vi "Dashboard Main.vi"() -> ()   [LabVIEW 2016]
uses:
  <vilib>/Utility/miscctls.llb/LVRowAndColumnTypeDef.ctl
  <vilib>/event_ctls.llb/eventvkey.ctl
  <vilib>/Rock Robotics/Network Tables/NT Read Numeric Array.vi
  <vilib>/Rock Robotics/WPI/Dashboard/WPI_DashboardLogging Global.vi
panel:
  in  "Camera Settings Right":T1={"Frame Rate"=30, "Compression"=30, "Size"=1, "DB Camera Config"=FALSE} {"Frame Rate" scale=1.0..30.0; "Compression" scale=100.0..-1.0; "Size" items=["640x480", "320x240", "160x120"]}
  in  "Camera Name Right":string(combo)="No Camera Selection"
  out "Camera Info":cluster{"Mbps LED":bool, "Mbps":dbl, "fps":dbl} {"fps" format="%#.1g"; "Mbps" format="%#.1g"}
  in  "Camera Settings":T1={"Frame Rate"=30, "Compression"=30, "Size"=1, "DB Camera Config"=FALSE} {"Frame Rate" scale=1.0..30.0; "Compression" scale=100.0..-1.0; "Size" items=["640x480", "320x240", "160x120"]}
  in  "TCP":refnum<k5>
  in  "Rec Mode":enum32{"Stop", "Record", "Playback"}(radio)
  out "Robot IP":string
  out "Image Message":string="Timeout in Camera Communications"
  in  "Dashboard Tab":T2(tab)
  in  "Select Auto":string(combo)="Select Autonomous ..."
  out "NT Connection":bool
  out "MotorChart R":cluster{"Numeric":dbl, "Numeric":dbl}(graph)
  out "MotorChart L":cluster{"Numeric":dbl, "Numeric":dbl}(graph)
  out "MotorSliders R":cluster{"MotorSlide1":dbl, "MotorSlide2":dbl} {"MotorSlide2" scale=-1.0..1.0 scale format="%#_2e"; "MotorSlide1" scale=-1.0..1.0 scale format="%#_2e"}
  out "MotorSliders L":cluster{"MotorSlide1":dbl, "MotorSlide2":dbl} {"MotorSlide2" scale=-1.0..1.0 scale format="%#_2e"; "MotorSlide1" scale=-1.0..1.0 scale format="%#_2e"}
  out "Gyro":dbl(knob) scale=0.0..360.0
  out "JS1 Z":dbl(slide) scale=-1.0..1.0 scale format="%#_2e"
  out "JS1 Graph":cluster{"X":dbl, "Y":dbl}[](graph)
  out "JS1 Buttons":T3
  out "JS2 Z":dbl(slide) scale=-1.0..1.0 scale format="%#_2e"
  out "JS2 Graph":cluster{"X":dbl, "Y":dbl}[](graph)
  out "JS2 Buttons":T3
  out "Mode":T4(ring)=enum."Auto Disabled"
  out "Camera Image Right":T5(plugin-control)
  in  "DB/String 9":string
  in  "DB/String 8":string
  in  "DB/String 7":string
  in  "DB/String 6":string
  in  "DB/String 5":string
  in  "DB/String 4":string
  in  "DB/String 3":string
  in  "DB/String 2":string
  in  "DB/String 1":string
  in  "DB/String 0":string
  in  "DB/Slider 0":dbl(slide) scale=0.0..5.0
  in  "DB/Slider 1":dbl(slide) scale=0.0..5.0
  in  "DB/Slider 2":dbl(slide) scale=0.0..5.0
  in  "DB/Slider 3":dbl(slide) scale=0.0..5.0
  out "DB/LED 3":bool
  out "DB/LED 2":bool
  out "DB/LED 1":bool
  out "DB/LED 0":bool
  in  "DB/Button 3":bool
  in  "DB/Button 2":bool
  in  "DB/Button 1":bool
  in  "DB/Button 0":bool caption="New Name"
  in  "JoystickModes":u16(ring)=3 items=["Arcade Joystick", "Tank", "Xbox top", "Xbox Right"]
  in  "Test Slider":dbl(slide) scale=0.0..100.0 scale format="%#_3g"
  in  "On/Off":bool caption="Solenoid"
  in  "Test Name":u16(ring) items=["Select the test to run..."]
  in  "Test Tree":string(tree)
  in  "Motor":cluster{"Value":dbl, "Enable":bool} {"Value" scale=-1.0..1.0 scale format="%#_3g"}
  out "Progress":T6 {"Test Progress" scale=0.0..100.0}
  in  "Rev/Fwd":cluster{"Forward":bool, "Reverse":bool}
  in  "Test Ring":u16(ring) items=["Monochrome", "Color"]
  out "Cmd Status":string
  in  "Execute Command":bool
  in  "Command Params":string[][](table)
  in  "Command Selection":i32(listbox)
  in  "CheckList":i32(listbox)
  out "Tree":string(tree)
  out "Camera Image":T5(plugin-control)
  out "Background":bool
  in  "Camera Name":string(combo)="No Camera Selection"
  # "HW"
  # "HW"
  # "Joysticks"
  # "Drive Motors"
  # "Front"
  # "Right"
  # "Left"
  # "Back"
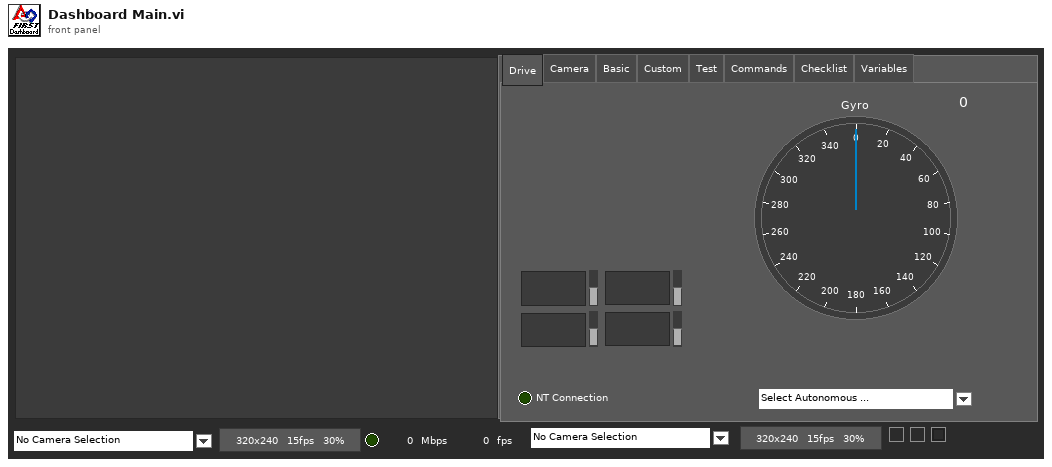
[diagram p1: front panel]
types:
  T1 = cluster{"Frame Rate":i32, "Compression":i32, "Size":u16, "DB Camera Config":bool}
  T2 = enum32{"Drive", "Camera", "Basic", "Custom", "Test", "Commands", "Checklist", "Variables"}
  T3 = cluster{bool, bool, bool, bool, bool, bool, bool, bool, bool, bool, bool, bool}
  T4 = enum8{"Tele-Op Disabled", "Tele-Op Enabled", "Auto Disabled", "Auto Enabled", "Test Disabled", "Test Enabled", "Disconnected", "No Code", "E-Stop"}
  T5 = typedef "IMAQ Image.ctl" = refnum<image>
  T6 = cluster{"Test Progress":u8, "Test Progress Text":string}
  T7 = typedef "Image Type" = u32
  T8 = cluster{"IDs":cluster{"RPC field ID":u16, "Unique ID":u16}, "String":string}
  T9 = enum32{"Drive", "Basic", "Custom", "Test", "Checklist", "Variables"}
  T10 = cluster{"Error Strings":string, "Disable Counts":cluster{u16, u16}, "Rail Faults":cluster{u16, u16, u16}, "Robot IP":string, "DB Mode":u8, "Event Info":cluster{"Name":string, "Type":u8, "Number":u16, "Replay":u8}}
  T11 = cluster{"Storage":cluster{"Disk Free":u64, "RAM Block":u32, "RAM free":u32}, "CPU Utilization":cluster{"CPU % ISR":sgl, "CPU % Time Crit":sgl, "CPU % Timed Str":sgl, "CPU % High":sgl, "CPU % Above":sgl, "CPU % Normal":sgl, "CPU % Low":sgl}, "CAN":cluster{"% Bus Utilization":sgl, "Bus Off Cnt":u32, "TX_FIFO Full Cnt":u32, "Receive Error Cnt":u8, "Transmit Error Cnt":u8}, "HID":cluster{"HID Outputs":u32, "Rumble Low":u16, "Rumble High":u16}[]}
  T12 = cluster{"Status bits":cluster{"Test Mode":bool, "Autonomous":bool, "Enabled":bool, "Code Start":bool, "Brownout":bool, "Reserved 2":bool, "Reserved 3":bool, "E-Stop":bool}, "Code Trace":cluster{"Disabled":bool, "TeleOp":bool, "Auto":bool, "Test":bool}, "Controller Type":enum16{"unknown", "cRIO", "roboRio"}, "Code?":enum16{"unknown", "noCode", "code"}, "Battery V":dbl}
  T13 = cluster{"Control Bits":cluster{"TestMode":bool, "Autonomous":bool, "Enabled":bool, "FMS Present":bool, bool, bool, bool, "E-Stop":bool}, "Team Station ":u8, "Countdown":sgl, "Joystick Values":cluster{"Axes":dbl[], "Buttons":bool[], "POVs":i16[]}[]}
  T14 = cluster{"Axes":dbl[], "Buttons":bool[], "POVs":i16[]}[]
  T15 = cluster{"Axes":dbl[], "Buttons":bool[], "POVs":i16[]}
  T16 = cluster{"Buttons[0]":bool, "Buttons[1]":bool, "Buttons[2]":bool, "Buttons[3]":bool, "Buttons[4]":bool, "Buttons[5]":bool, "Buttons[6]":bool, "Buttons[7]":bool, "Buttons[8]":bool, "Buttons[9]":bool, "Buttons[10]":bool, "Buttons[11]":bool}
  T17 = cluster{"Camera Image":refnum<vi>, "Dashboard Tab":refnum<vi>, "Background":refnum<vi>, "Rec Mode":refnum<vi>, "Test Slider":refnum<vi>, "On/Off ":refnum<vi>, "Test Ring":refnum<vi>, "Rev/Fwd":refnum<vi>, "Test Name":refnum<vi>, "Motor":refnum<vi>, "Progress":refnum<vi>, "CheckList":refnum<vi>, "Tree":refnum<vi>, "Test Tree":refnum<vi>, "Command Params":refnum<vi>, "Command Selection":refnum<vi>, "Execute Command":refnum<vi>, "Cmd Status":refnum<vi>, "Camera Settings":refnum<vi>, "Camera Name":refnum<vi>, "Camera Info":refnum<vi>, "Camera Settings Right":refnum<vi>, "Camera Name Right":refnum<vi>, "Camera Image Right":refnum<vi>}
  T18 = cluster{"Operation":enum16{"Update", "Clear"}, "Color Box":u32}[]
  T19 = typedef "eventvkey.ctl" = enum16{"ASCII", "Enter", "Return", "Shift", "Ctrl", "Alt", "Cmd", "Opt", "Caps", "NumLock", "Clear", "Break", "Up", "Down", "Left", "Right", "Insert", "Delete", "Home", "End", "PageUp", "PageDown", "Escape", "Help", "Pause", "ScrollLock", "F1", "F2", "F3", "F4", "F5", "F6", "F7", "F8", "F9", "F10", "F11", "F12", "F13", "F14", "F15", "F16", "F17", "F18", "F19", "F20", "F21", "F22", "F23", "F24", "Play", "VolumeUp", "VolumeDown", "Mute", "Two Byte Char"}
  T20 = cluster{"Image Size":bool, "Image Type":bool, "Pixel Value":bool, "ROI Information":bool, "Zoom Factor":bool}
  T21 = cluster{"Operation":enum16{"Update", "Clear"}, "Color Box":u32}
  T22 = typedef "LVRowAndColumnTypeDef.ctl" = cluster{"Row":i32, "Column":i32}
  T23 = cluster{"Shift":bool, "Ctrl":bool, "Alt":bool, "Cmd":bool, "Opt":bool}
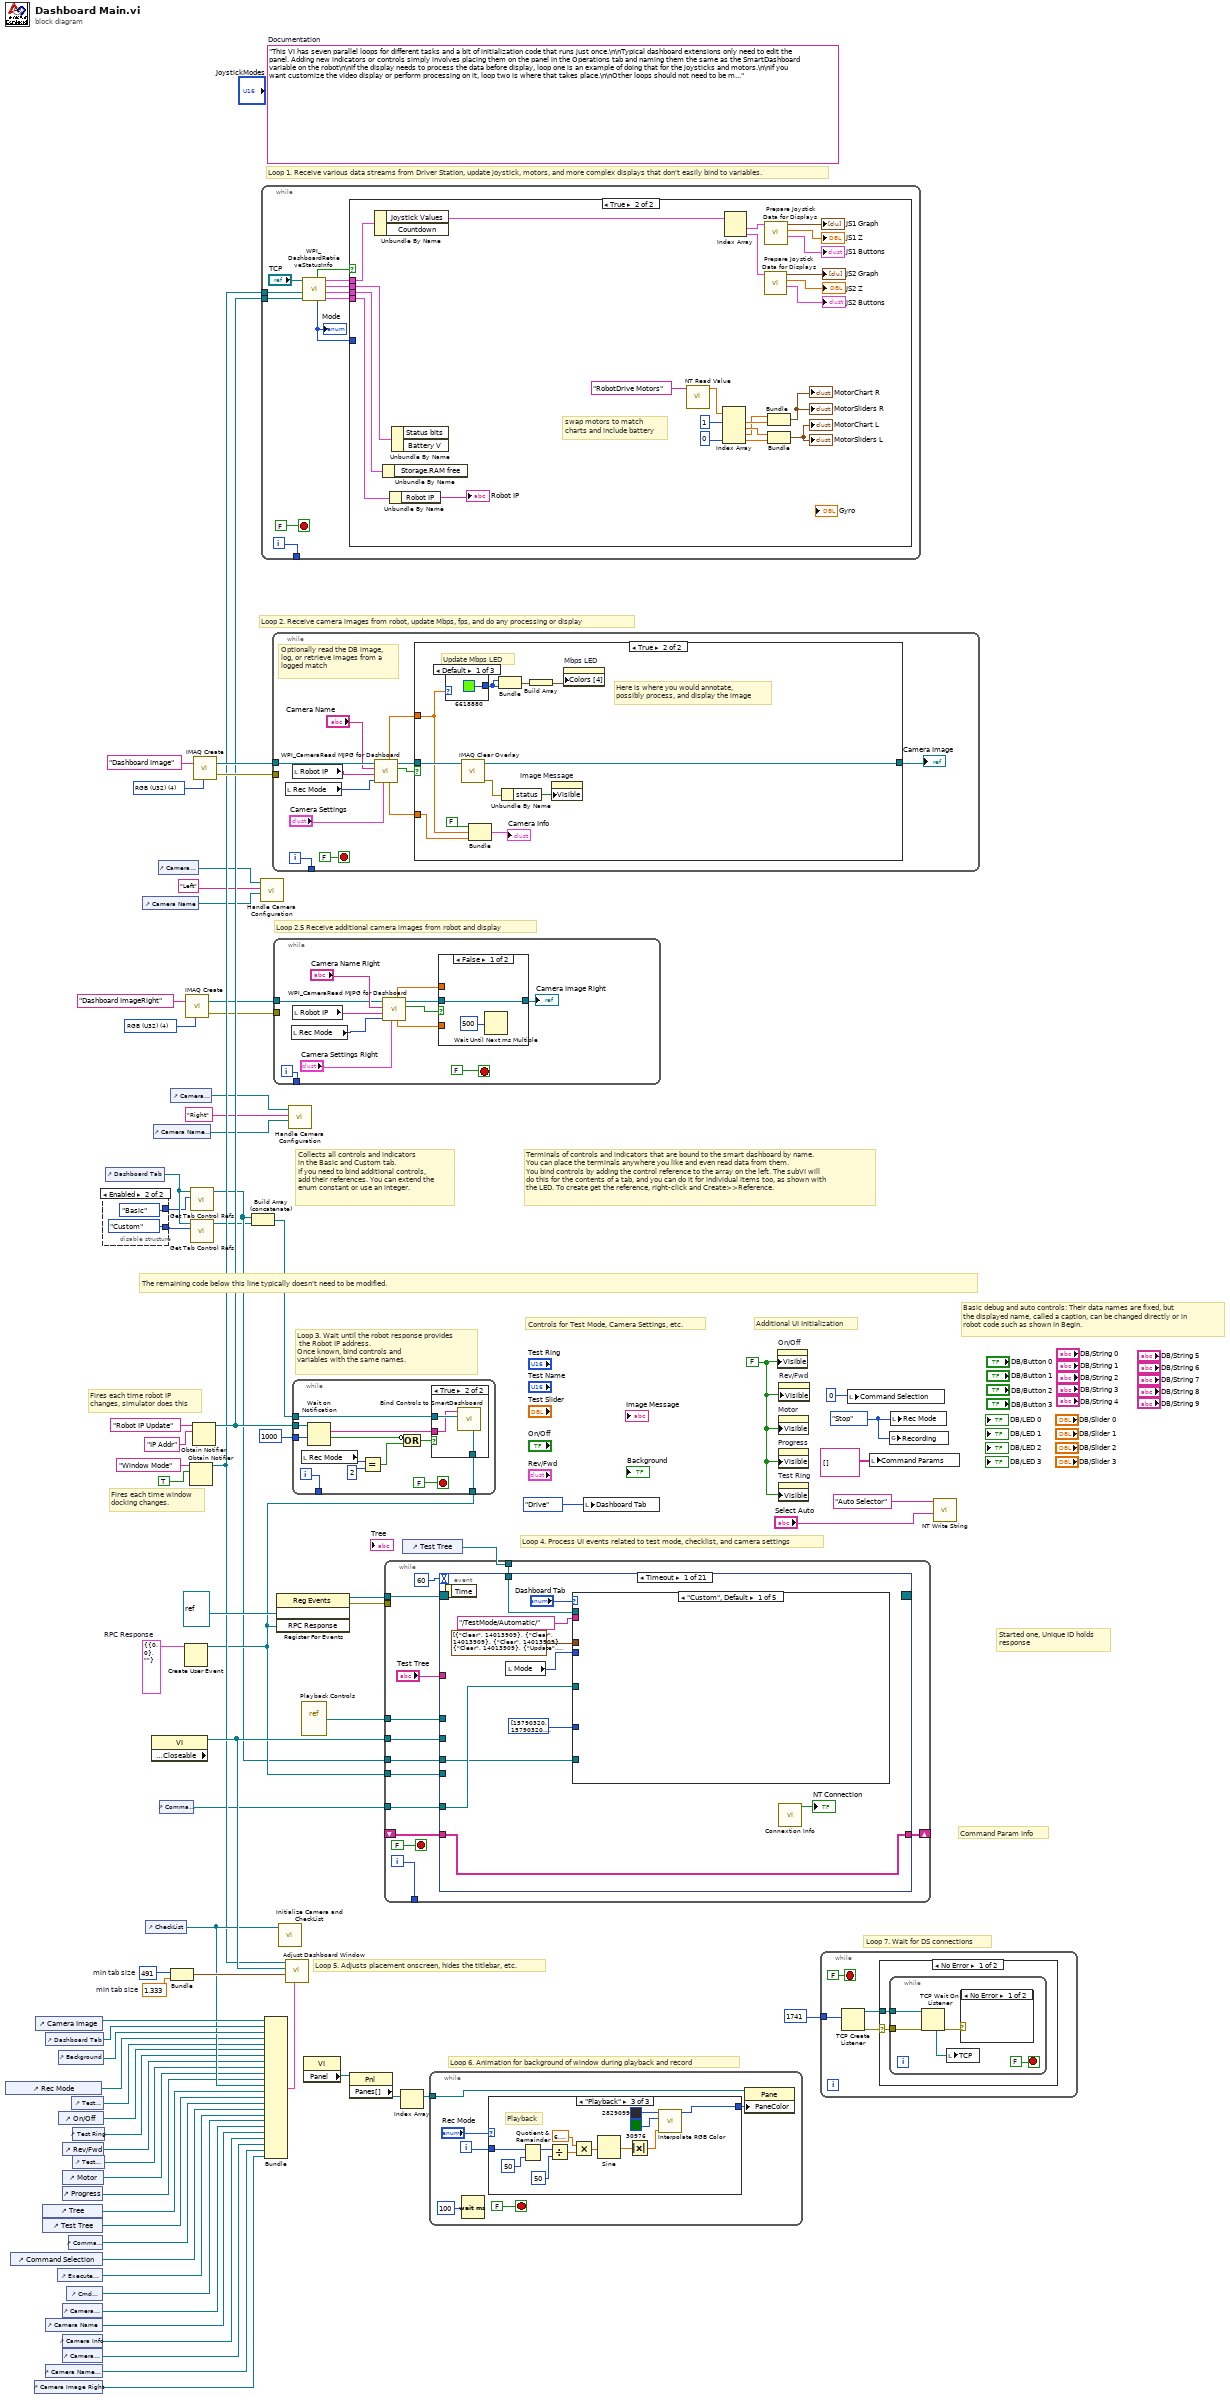
[diagram p0: block diagram]
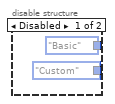
[diagram p2: hidden frame]
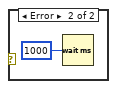
[diagram p4: hidden frame]
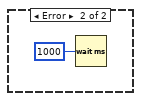
[diagram p5: hidden frame]
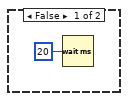
[diagram p6: hidden frame]
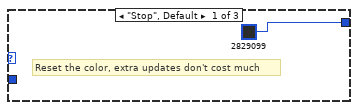
[diagram p7: hidden frame]
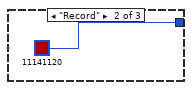
[diagram p8: hidden frame]
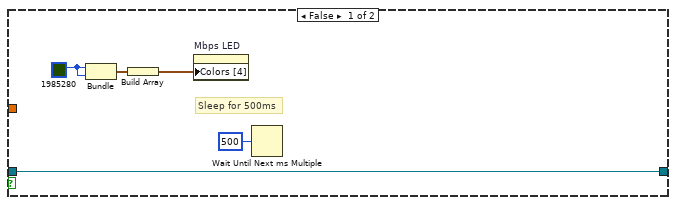
[diagram p10: hidden frame]
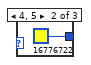
[diagram p11: hidden frame]
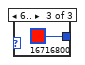
[diagram p12: hidden frame]
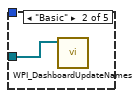
[diagram p13: hidden frame]
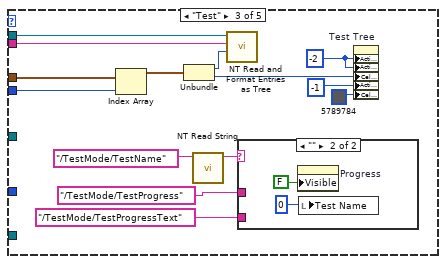
[diagram p14: hidden frame]
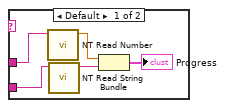
[diagram p15: hidden frame]
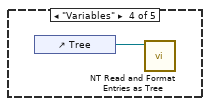
[diagram p16: hidden frame]
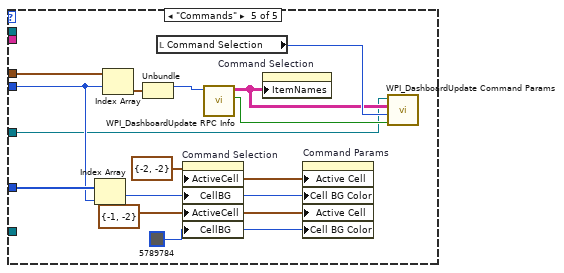
[diagram p17: hidden frame]
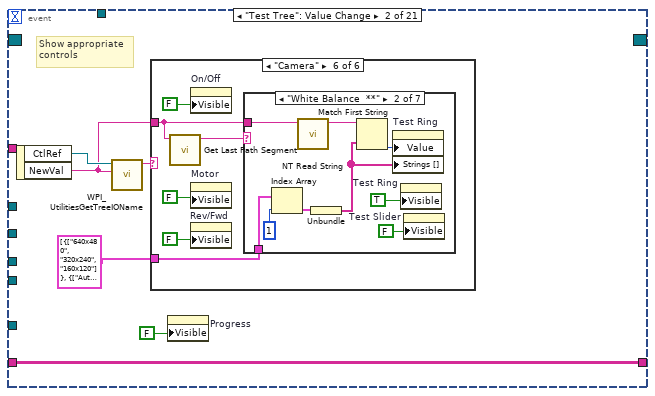
[diagram p18: hidden frame]
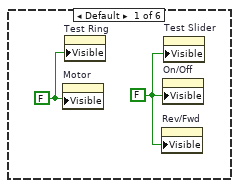
[diagram p19: hidden frame]
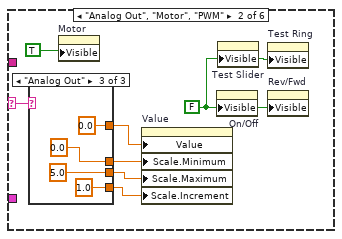
[diagram p20: hidden frame]
diagram:
  w12 = T7 4 items=["Grayscale (U8)", "Grayscale (I16)", "Grayscale (SGL)", "Complex (CSG)", "RGB (U32)", "HSL (U32)", "RGB (U64)"] ("Image Type")
  w27 = T8 {"IDs"={"RPC field ID"=0, "Unique ID"=0}, "String"=""}  # RPC Response
  w52 = 491  # min tab size
  w51 = 1.333  # min tab size
  w58 = enum32{"Stop", "Record", "Playback"}."Stop" ("Rec Mode")
  w34 = FALSE ("Visible")
  (unwired) "This VI has seven parallel loops for different tasks and a bit of initialization code that runs just once.\n\nTypical dashboard extensions only need to edit the panel. Adding new indicators or controls simply involves placing them on the panel in the Operations tab and naming them the same as the SmartDashboard variable on the robot\n\nIf the display needs to process the data before display, loop one is an example of doing that for the joysticks and motors.\n\nIf you want customize the video display or perform processing on it, loop two is where that takes place.\n\nOther loops should not need to be modified. They are pretty standard, and document the task they perform."  # Documentation
  w75 = T7 4 items=["Grayscale (U8)", "Grayscale (I16)", "Grayscale (SGL)", "Complex (CSG)", "RGB (U32)", "HSL (U32)", "RGB (U64)"] ("Image Type")
  # "Loop 2.5 Receive additional camera images from robot and display"
  # "Command Param Info"
  # "Started one, Unique ID holds\nresponse"
  # "Loop 7. Wait for DS connections"
  # "Basic debug and auto controls: Their data names are fixed, but\nthe displayed name, called a caption, can be changed directly or in\nrobot code such as shown in Begin."
  # "Controls for Test Mode, Camera Settings, etc."
  # "Additional UI Initialization"
  # "Loop 6. Animation for background of window during playback and record"
  # "Fires each time robot IP\nchanges, simulator does this"
  # "Fires each time window\ndocking changes."
  # "Collects all controls and indicators\nin the Basic and Custom tab.\nIf you need to bind additional controls,\nadd their references. You can extend the\nenum constant or use an integer."
  # "The remaining code below this line typically doesn't need to be modified."
  # "Loop 4. Process UI events related to test mode, checklist, and camera settings"
  # "Terminals of controls and indicators that are bound to the smart dashboard by name.\nYou can place the terminals anywhere you like and even read data from them.\nYou bind controls by adding the control reference to the array on the left. The subVI will\ndo this for the contents of a tab, and you can do it for individual items too, as shown with\nthe LED. To create get the reference, right-click and Create>>Reference."
  # "Loop 3. Wait until the robot response provides\n the Robot IP address.\nOnce known, bind controls and\nvariables with the same names."
  # "Loop 5. Adjusts placement onscreen, hides the titlebar, etc."
  # "Loop 1. Receive various data streams from Driver Station, update joystick, motors, and more complex displays that don't easily bind to variables."
  # "Loop 2. Receive camera images from robot, update Mbps, fps, and do any processing or display"
  n1 = control-ref of="Rec Mode"() -> (w40:refnum<vi>)
  n2 = control-ref of="Command Selection"() -> (w26:refnum<vi>)
  n3 = control-ref of="Camera Image Right"() -> (w3:refnum<vi>)
  n4 = control-ref of="Camera Image"() -> (w54:refnum<vi>)
  n5 = control-ref of="Tree"() -> (w44:refnum<vi>)
  n6 = control-ref of="Test Tree"() -> (w43:refnum<vi>)
  n7 = control-ref of="Dashboard Tab"() -> (w53:refnum<vi>)
  n8 = control-ref of="Camera Name"() -> (w17:refnum<vi>)
  n9 = control-ref of="Camera Name Right"() -> (w4:refnum<vi>)
  n10 = control-ref of="Execute Command"() -> (w28:refnum<vi>)
  n11 = control-ref of="Background"() -> (w49:refnum<vi>)
  n12 = control-ref of="On/Off"() -> (w38:refnum<vi>)
  n13 = control-ref of="Progress"() -> (w35:refnum<vi>)
  n14 = control-ref of="Camera Settings"() -> (w18:refnum<vi>)
  n15 = control-ref of="Camera Info"() -> (w16:refnum<vi>)
  n16 = control-ref of="Camera Settings Right"() -> (w5:refnum<vi>)
  n17 = control-ref of="Rev/Fwd"() -> (w36:refnum<vi>)
  n18 = control-ref of="Motor"() -> (w41:refnum<vi>)
  n19 = control-ref of="Cmd Status"() -> (w22:refnum<vi>)
  n20 = control-ref of="Command Params"() -> (w29:refnum<vi>)
  n21 = control-ref of="Test Slider"() -> (w39:refnum<vi>)
  n22 = control-ref of="Test Ring"() -> (w37:refnum<vi>)
  n23 = control-ref of="Test Name"() -> (w42:refnum<vi>)
  n24 = disable-structure shown="Enabled" {
    disable-tunnel: [T9."Basic" ("Dashboard Tab") T2."Basic" ("Dashboard Tab")] -> w48
    disable-tunnel: [T9."Custom" ("Dashboard Tab") T2."Custom" ("Dashboard Tab")] -> w47
    frame Disabled {
    }
    frame Enabled {
    }
  }
  n25 = control-ref of="Dashboard Tab"() -> (w56:refnum<vi>)
  n26 = control-ref of="Camera Name"() -> (w19:refnum<vi>)
  n27 = control-ref of="CheckList"() -> (w45:refnum<vi>)
  n28 = property class="VI" props=["Front Panel.Closeable"]() -> (reference out=w57:refnum<vi>)  [unwired: 2 in, 2 out]
  n29 = control-ref of="Camera Name Right"() -> (w8:refnum<vi>)
  n30 = control-ref of="Camera Settings"() -> (w20:refnum<vi>)
  n31 = control-ref of="Command Params"() -> (w21:refnum<vi>)
  n32 = control-ref of="Camera Settings Right"() -> (w9:refnum<vi>)
  n33 = Bundle("min tab size"=w52, "min tab size"=w51) -> (w50:cluster{"min tab size":i32, "min tab size":dbl})  [unwired: 1 in]
  n34 = Create User Event(user event datatype=w27) -> (user event=w23:refnum<user-event>)  [unwired: 1 in, 1 out]
  n35 = call "IMAQ Create"("Image Name"="Dashboard ImageRight", "Image Type"=w12) -> ("New Image"=w11:T5, "error out"=w10:errorcluster)  [unwired: 2 in, 1 out]
  n36 = Obtain Notifier(name (unnamed)="Window Mode", notification data type=TRUE) -> (notifier out=w32:refnum<notifier>)  [unwired: 2 in, 2 out]
  n37 = call <vilib>:"Get Tab Control Refs.vi"("Page Index"=w48, "TabControl in"=w56) -> ("ControlsOnPage"=w2:refnum<vi>[])  [unwired: 9 in]
  n38 = call <vilib>:"Get Tab Control Refs.vi"("Page Index"=w47, "TabControl in"=w56) -> ("ControlsOnPage"=w1:refnum<vi>[])  [unwired: 9 in]
  n39 = Obtain Notifier(name (unnamed)="Robot IP Update", notification data type="IP Addr" ("name (unnamed)")) -> (notifier out=w33:refnum<notifier>)  [unwired: 2 in, 2 out]
  n40 = call "IMAQ Create"("Image Name"="Dashboard Image", "Image Type"=w75) -> ("New Image"=w73:T5, "error out"=w72:errorcluster)  [unwired: 2 in, 1 out]
  n41 = Build Array (concatenate)(w2, w1) -> (w55:refnum<vi>[])
  n42 = call "Handle Camera Configuration.vi"("CameraNameRef"=w19, "Camera File Name"="Left", "ClusterRef"=w20) -> ()  [unwired: 9 in]
  n43 = while {
    tunnel: [w89] -> _
    tunnel: w33 -> [w83]
    tunnel: w32 -> [w80]
    i -> [w89]
    stop <- FALSE stop-if-true
    n44 = call <vilib>:"WPI_DashboardRetrieveStatusInfo.vi"("Binding Refnum"=w83, "Window Mode Notifier"=w80, "TCP Cnx"="TCP") -> ("Power and Errors"=w84:T10, "Robot Metrics"=w87:T11, "Status Info"=w88:T12, "Control Info"=w85:T13, "Robot Mode"=w82:T4, "Process?"=w86:bool)  [unwired: 3 in]
    "Mode" <- w82
    n45 = case shown="True" w86 {
      tunnel: w88 -> [_ w115]
      tunnel: w87 -> [_ w114]
      tunnel: w85 -> [_ w113]
      tunnel: w84 -> [_ w112]
      tunnel: w82 -> [_ _]
      frame False {
        n46 = Wait (ms)(milliseconds to wait=u32 20) -> ()  [unwired: 1 out]
      }
      frame True {
        # "swap motors to match\ncharts and include battery"
        n47 = Unbundle By Name(w113) -> ("Joystick Values"=w103:T14)  [unwired: 1 out]
        n48 = Unbundle By Name(w114) -> ()  [unwired: 1 out]
        n49 = Unbundle By Name(w112) -> ("Robot IP"=→"Robot IP":string)
        n50 = Unbundle By Name(w115) -> ()  [unwired: 2 out]
        n51 = call-poly <vilib>:"NT Read Value.vi"("Name"="RobotDrive Motors") -> ("Numeric Array"=w93:dbl[])  [unwired: 9 in, 1 out]
        n52 = Index Array(array=w93, index #1=1, index #4=0) -> (element #1=w107:dbl, element #2=w108:dbl, element #3=w106:dbl, element #4=w111:dbl)  [unwired: 2 in]
        n53 = Index Array(array=w103) -> (element #1=w102:T15, element #2=w98:T15)  [unwired: 2 in]
        n54 = call "Prepare Joystick Data for Displays.vi"("Joystick Values"=w98) -> ("Buttons"=→"JS2 Buttons":T16, "Z Axis"=→"JS2 Z":dbl, "Cartesian Data"=→"JS2 Graph":cluster{"X axis":dbl, "X axis":dbl}[])  [unwired: 8 in]
        n55 = call "Prepare Joystick Data for Displays.vi"("Joystick Values"=w102) -> ("Buttons"=→"JS1 Buttons":T16, "Z Axis"=→"JS1 Z":dbl, "Cartesian Data"=→"JS1 Graph":cluster{"X axis":dbl, "X axis":dbl}[])  [unwired: 8 in]
        n56 = Bundle("Numeric"=w106, "Numeric"=w107) -> (→"MotorChart R" →"MotorSliders R":cluster{"Numeric":dbl, "Numeric":dbl})  [unwired: 1 in]
        n57 = Bundle("Numeric"=w108, "Numeric"=w111) -> (→"MotorChart L" →"MotorSliders L":cluster{"Numeric":dbl, "Numeric":dbl})  [unwired: 1 in]
      }
    }
  }
  n58 = Bundle("Camera Image"=w54, "Dashboard Tab"=w53, "Background"=w49, "Rec Mode"=w40, "Test Slider"=w39, "On/Off"=w38, "Test Ring"=w37, "Rev/Fwd"=w36, "Test Name"=w42, "Motor"=w41, "Progress"=w35, "CheckList"=w45, "Tree"=w44, "Test Tree"=w43, "Command Params"=w29, "Command Selection"=w26, "Execute Command"=w28, "Cmd Status"=w22, "Camera Settings"=w18, "Camera Name"=w17, "Camera Info"=w16, "Camera Settings Right"=w5, "Camera Name Right"=w4, "Camera Image Right"=w3) -> (w46:T17)  [unwired: 1 in]
  n59 = while {
    tunnel: w73 -> [w125]
    tunnel: w72 -> [_]
    tunnel: [w126] -> _
    i -> [w126]
    stop <- FALSE stop-if-true
    # "Optionally read the DB image,\nlog, or retrieve images from a\nlogged match"
    n60 = local read "Rec Mode"() -> (w121:enum32{"Stop", "Record", "Playback"})
    n61 = local read "Robot IP"() -> (w120:string)
    n62 = call <vilib>:"WPI_CameraRead MJPG for Dashboard.vi"("Camera Settings"="Camera Settings", "Rec Mode"=w121, "Robot IP"=w120, "Camera Name"="Camera Name", "Refnum in"=w125) -> ("Active"=w123:bool, "Refnum out"=w124:T5, "FPS"=w122:dbl, "Bandwidth (Mbps)"=w119:dbl)  [unwired: 3 in]
    n63 = case shown="True" w123 {
      tunnel: w124 -> [w128 w139]
      tunnel: w119 -> [_ w136]
      tunnel: w122 -> [_ w137]
      tunnel: [w128 w133] -> w116
      frame False {
        w130 = u32 1985280 ("Color Box")
        # "Sleep for 500ms"
        n64 = Bundle("Color Box"=w130, "Color Box"=w130) -> (w131:cluster{"Color Box":u32, "Color Box":u32})  [unwired: 1 out]
        n65 = Build Array(w131) -> (w129:cluster{"Color Box":u32, "Color Box":u32}[])
        n66 = property on="Mbps LED" class="Bool (strict)"("Colors [4]"=w129) -> ()  [unwired: 2 in, 2 out]
        n67 = Wait Until Next ms Multiple(millisecond multiple=u32 500) -> ()  [unwired: 1 out]
      }
      frame True {
        # "Here is where you would annotate,\npossibly process, and display the image"
        # "Update Mbps LED"
        n68 = case shown="Default" w136 {
          tunnel: [u32 6618880 ("Color Box") u32 16776722 ("Color Box") u32 16716800 ("Color Box")] -> w140
          frame Default {
          }
          frame 4, 5 {
          }
          frame 6.. {
          }
        }
        n69 = call "IMAQ Clear Overlay"("Image"=w139) -> ("error out"=w142:errorcluster, "Image Out"=w133:T5)  [unwired: 2 in, 7 out]
        n70 = Bundle(FALSE, "Bandwidth (Mbps)"=w136, "FPS"=w137) -> (→"Camera Info":cluster{bool, "Bandwidth (Mbps)":dbl, "FPS":dbl})  [unwired: 1 in]
        n71 = Bundle("Color Box"=w140, "Color Box"=w140) -> (w141:cluster{"Color Box":u32, "Color Box":u32})  [unwired: 1 out]
        n72 = Unbundle By Name(w142) -> ("status"=w143:bool)
        n73 = Build Array(w141) -> (w138:cluster{"Color Box":u32, "Color Box":u32}[])
        n74 = property on="Image Message" class="Str"("Visible"=w143) -> ()  [unwired: 2 in, 2 out]
        n75 = property on="Mbps LED" class="Bool (strict)"("Colors [4]"=w138) -> ()  [unwired: 2 in, 2 out]
      }
    }
    "Camera Image" <- w116
  }
  n76 = while {
    tunnel: w11 -> [w157]
    tunnel: w10 -> [_]
    tunnel: [w151] -> _
    i -> [w151]
    stop <- FALSE stop-if-true
    n77 = local read "Rec Mode"() -> (w155:enum32{"Stop", "Record", "Playback"})
    n78 = local read "Robot IP"() -> (w156:string)
    n79 = call <vilib>:"WPI_CameraRead MJPG for Dashboard.vi"("Camera Settings"="Camera Settings Right", "Rec Mode"=w155, "Robot IP"=w156, "Camera Name"="Camera Name Right", "Refnum in"=w157) -> ("Active"=w150:bool, "Refnum out"=w153:T5, "FPS"=w148:dbl, "Bandwidth (Mbps)"=w149:dbl)  [unwired: 3 in]
    n80 = case shown="False" w150 {
      tunnel: w153 -> [w159 w161]
      tunnel: w149 -> [_ _]
      tunnel: w148 -> [_ _]
      tunnel: [w159 w161] -> w147
      frame False {
        n81 = Wait Until Next ms Multiple(millisecond multiple=u32 500) -> ()  [unwired: 1 out]
      }
      frame True {
      }
    }
    "Camera Image Right" <- w147
  }
  n82 = register-events(refnum<vi> refnum, w23) -> (reference out=w62:refnum<event-registration>, error out=w61:errorcluster)  [unwired: 2 in]
  n83 = call "Initialize Camera and CheckList.vi"("ListBox in"=w45) -> ()  [unwired: 11 in]
  n84 = call "Adjust Dashboard Window.vi"("Sizing Refnums"=w46, "Size Constraints"=w50, "VI"=w57, "WIn Mode"=w32) -> ()  [unwired: 8 in]
  n85 = call "Handle Camera Configuration.vi"("CameraNameRef"=w8, "Camera File Name"="Right", "ClusterRef"=w9) -> ()  [unwired: 9 in]
  n86 = while {
    tunnel: w55 -> [w173]
    tunnel: w33 -> [w171]
    tunnel: [w169] -> _
    tunnel: u32 1000 ("milliseconds to wait") -> [w168]
    tunnel: w23 -> [w162]
    i -> [w169]
    stop <- FALSE stop-if-true
    n87 = local read "Rec Mode"() -> (w164:enum32{"Stop", "Record", "Playback"})
    n88 = Wait on Notification(notifier=w171, timeout in ms (-1)=w168) -> (notification=w170:string, timed out?=w166:bool)  [unwired: 2 in, 2 out]
    n89 = Equal?(x=w164, y=u16 2 ("Rec Mode")) -> (x = y?=w165:bool)
    n90 = Compound Arithmetic op=OR(invert w166, w165) -> (w167:bool)
    n91 = case shown="True" w167 {
      tunnel: w173 -> [_ w176]
      tunnel: w170 -> [_ w175]
      tunnel: w162 -> [_ w174]
      frame False {
      }
      frame True {
        n92 = call <vilib>:"Bind Controls to SmartDashboard.vi"("RPC ref"=w174, "Bound Control Refs"=w176, "Server IP Address"=w175) -> ()  [unwired: 9 in]
      }
    }
  }
  n93 = vi-ref "Playback Controls.vi"() -> (w63:refnum<vi>)
  n94 = property class="VI"() -> ("Panel"=w65:refnum<vi>)  [unwired: 2 in, 2 out]
  n95 = property class="Pnl"(reference=w65) -> ("Panes[]"=w66:refnum<vi>[])  [unwired: 1 in, 2 out]
  n96 = Index Array(array=w66) -> (element=w64:refnum<vi>)  [unwired: 1 in]
  n97 = control-ref of="Test Tree"() -> (w67:refnum<vi>)
  n98 = while {
    tunnel: [w186] -> _
    tunnel: w67 -> [w185]
    tunnel: w63 -> [w184]
    tunnel: w62 -> [w183]
    tunnel: w61 -> [_]
    tunnel: w57 -> [w182]
    tunnel: w23 -> [w181]
    tunnel: w21 -> [w180]
    shift-right: [w179] -> _
    shift-left: _ -> [w178]
    tunnel: w2 -> [w177]
    i -> [w186]
    stop <- FALSE stop-if-true
    n99 = event shown="[0] Timeout" {
      selector: w183 -> [_ _ _ _ _ _ _ _ _ _ _ _ _ _ _ _ _ _ _ _ _]
      dyn-events: [_ _ _ _ _ _ _ _ _ _ _ _ _ _ _ _ w442 _ _ _ _] -> _
      timeout: u32 60 ("milliseconds to wait") -> [_ _ _ _ _ _ _ _ _ _ _ _ _ _ _ _ _ _ _ _ _]
      tunnel: w185 -> [w198 _ _ _ _ _ _ _ _ _ _ _ _ _ _ _ _ _ _ _ _]
      tunnel: "Test Tree" -> [_ _ _ _ _ _ _ _ _ _ _ w409 w417 w419 w423 w431 _ _ _ _ _]
      tunnel: w184 -> [_ _ _ _ _ _ _ _ _ _ _ _ _ _ _ _ w444 _ w462 _ _]
      tunnel: w182 -> [_ _ _ _ _ _ _ _ _ _ _ _ _ _ _ _ w440 _ _ _ _]
      tunnel: w181 -> [_ _ _ _ _ _ _ _ _ _ _ _ _ _ _ _ w436 _ _ _ _]
      tunnel: w180 -> [w193 _ _ _ _ _ w360 _ _ _ _ _ _ _ _ _ _ _ _ _ _]
      tunnel: [w192 w237 w339 w344 w353 w357 w358 w367 w377 w384 w396 w408 w415 w418 w422 w430 w435 w457 w459 w463 w474] -> w179
      tunnel: w178 -> [w192 w237 w339 w344 w353 w357 w358 _ _ w384 w396 w408 w415 w418 w422 w430 w435 w457 w459 w463 w474]
      tunnel: w177 -> [w190 _ _ _ _ _ _ _ _ _ _ _ _ _ _ _ _ _ _ _ _]
      event Timeout {
        n100 = event-data() -> ()  [unwired: 1 in, 1 out]
        n101 = local read "Mode"() -> (w195:T4)
        n102 = case shown="\"Custom\", Default" "Dashboard Tab" {
          tunnel: w198 -> [_ _ w214 _ _]
          tunnel: "/TestMode/Automatic/" ("Name Pattern") -> [_ _ w213 _ _]
          tunnel: T18 [{"Operation"=enum."Clear", "Color Box"=14013909}, {"Operation"=enum."Clear", "Color Box"=14013909}, {"Operation"=enum."Clear", "Color Box"=14013909}, {"Operation"=enum."Clear", "Color Box"=14013909}, {"Operation"=enum."Update", "Color Box"=14013909}, {"Operation"=enum."Update", "Color Box"=16777215}, {"Operation"=enum."Clear", "Color Box"=14013909}, {"Operation"=enum."Clear", "Color Box"=14013909}, {"Operation"=enum."Clear", "Color Box"=14013909}] -> [_ _ w206 _ w230]
          tunnel: w195 -> [_ _ w205 _ w229]
          tunnel: u32[] [15790320, 15790320, 15790320, 15790320, 16777215, 16777215, 15790320, 15790320, 15790320] -> [_ _ _ _ w235]
          tunnel: w193 -> [_ _ _ _ w223]
          tunnel: w190 -> [_ w200 _ _ _]
          frame "Custom", Default {
          }
          frame "Basic" {
            n103 = call <vilib>:"WPI_DashboardUpdateNames.vi"("Controls on Tab"=w200) -> ()  [unwired: 11 in]
          }
          frame "Test" {
            w212 = -2 ("Active Item:Row Number")
            n104 = Index Array(array=w206, index=w205) -> (element=w207:T21)
            n105 = Unbundle(w207) -> ("Operation"=w208:enum16{"Update", "Clear"}, "Color Box"=w209:u32)
            n106 = call <vilib>:"NT Read String.vi"("Name"="/TestMode/TestName") -> ("String"=w203:string)  [unwired: 9 in, 1 out]
            n107 = call <vilib>:"NT Read and Format Entries as Tree.vi"("Operation"=w208, "Name Pattern"=w213, "Tree Refnum"=w214) -> ()  [unwired: 7 in, 2 out]
            n108 = case shown="\"\"" w203 {
              tunnel: "/TestMode/TestProgress" ("Name") -> [w216 _]
              tunnel: "/TestMode/TestProgressText" ("Name") -> [w215 _]
              frame Default {
                n109 = call <vilib>:"NT Read Number.vi"("Name"=w216) -> ("Numeric"=w217:dbl)  [unwired: 9 in, 1 out]
                n110 = call <vilib>:"NT Read String.vi"("Name"=w215) -> ("String"=w218:string)  [unwired: 9 in, 1 out]
                n111 = Bundle("Numeric"=w217, "String"=w218) -> (→"Progress":cluster{"Numeric":dbl, "String":string})  [unwired: 1 in]
              }
              frame "" {
                n112 = property on="Progress" class="Clust (strict)"("Visible"=FALSE) -> ()  [unwired: 2 in, 2 out]
                n113 = local write "Test Name"(u16 0) -> ()
              }
            }
            n114 = property on="Test Tree" class="Tree (strict)"("Active Item Row Number"=w212, "ActiveColNum"=w212, "CellBG"=w209, "Active Item Row Number"=-1 ("Active Item:Row Number"), "CellBG"=u32 5789784 ("Color Box")) -> ()  [unwired: 2 in, 2 out]
          }
          frame "Variables" {
            n115 = control-ref of="Tree"() -> (w222:refnum<vi>)
            n116 = call <vilib>:"NT Read and Format Entries as Tree.vi"("Tree Refnum"=w222) -> ()  [unwired: 9 in, 2 out]
          }
          frame "Commands" {
            w231 = u32 5789784 ("Color Box")
            w232 = T22 {"Row"=-1, "Column"=-2} ("Active Cell:Active Cell")
            w234 = T22 {"Row"=-2, "Column"=-2} ("Active Cell:Active Cell")
            n117 = Index Array(array=w235, index=w229) -> (element=w233:u32)
            n118 = Index Array(array=w230, index=w229) -> (element=w228:T21)
            n119 = Unbundle(w228) -> ("Operation"=w227:enum16{"Update", "Clear"})  [unwired: 1 out]
            n120 = local read "Command Selection"() -> (w226:i32)
            n121 = property on="Command Selection" class="MCListbox (strict)"("ActiveCell"=w234, "CellBG"=w233, "ActiveCell"=w232, "CellBG"=w231) -> ()  [unwired: 2 in, 2 out]
            n122 = call <vilib>:"WPI_DashboardUpdate RPC Info.vi"("Operation"=w227) -> ("update"=w225:bool, "commands"=w224:string[][])  [unwired: 9 in]
            n123 = property on="Command Selection" class="MCListbox (strict)"("ItemNames"=w224) -> ()  [unwired: 2 in, 2 out]
            n124 = property on="Command Params" class="Tbl (strict)"("Active Cell"=w234, "Cell BG Color"=w233, "Active Cell"=w232, "Cell BG Color"=w231) -> ()  [unwired: 2 in, 2 out]
            n125 = call <vilib>:"WPI_DashboardUpdate Command Params.vi"("Update"=w225, "NewVal"=w226, "Commands"=w224, "Param Tbl"=w223) -> ()  [unwired: 7 in, 1 out]
          }
        }
        n126 = call <vilib>:"Connextion Info.vi"() -> ("Connected"=→"NT Connection":bool)  [unwired: 10 in, 1 out]
      }
      event "Test Tree": Value Change {
        # "Show appropriate\ncontrols"
        n127 = event-data() -> ("CtlRef"=w240:refnum<vi>, "NewVal"=w238:string)  [unwired: 1 in]
        n128 = call <vilib>:"WPI_UtilitiesGetTreeIOName.vi"("NewVal"=w238, "TreeControl in"=w240) -> ("I/O Name"=w241:string)  [unwired: 9 in]
        n129 = case shown="\"Camera\"" w241 {
          selector: w241 -> [_ w248 _ w270 w279 _]
          tunnel: w238 -> [_ _ w267 w269 _ w286]
          tunnel: cluster{string[]}[] [{["640x480", "320x240", "160x120"]}, {["Auto", "Fixed indoor", "Fixed outdoor 1", "Fixed outdoor 2", "Fixed fluorescent 1", "Fixed fluorescent 2", "Hold current"]}, {["Auto", "Flicker-free 50 Hz", "Flicker-free 60 Hz", "Hold current"]}, {["None", "Prioritize frame rate", "Prioritize image quality"]}, {["Monochrome", "Color"]}] -> [_ _ _ _ _ w285]
          frame Default {
            w243 = FALSE ("Visible")
            w242 = FALSE ("Visible")
            n130 = property on="Motor" class="Clust (strict)"("Visible"=w242) -> ()  [unwired: 2 in, 2 out]
            n131 = property on="Test Ring" class="Ring (strict)"("Visible"=w242) -> ()  [unwired: 2 in, 2 out]
            n132 = property on="Rev/Fwd" class="Clust (strict)"("Visible"=w243) -> ()  [unwired: 2 in, 2 out]
            n133 = property on="On/Off" class="Bool (strict)"("Visible"=w243) -> ()  [unwired: 2 in, 2 out]
            n134 = property on="Test Slider" class="Slide (strict)"("Visible"=w243) -> ()  [unwired: 2 in, 2 out]
          }
          frame "Analog Out", "Motor", "PWM" {
            w249 = FALSE ("Visible")
            n135 = case shown="\"Analog Out\"" w248 {
              tunnel: [1.0 ("Value") -1.0 ("Value") 0.0 ("Value")] -> w247
              tunnel: [255.0 ("Value") 1.0 ("Value") 5.0 ("Value")] -> w246
              tunnel: [128.0 ("Value") 0.0 ("Value") 0.0 ("Value")] -> w245
              tunnel: [64.0 ("Value") 0.5 ("Value") 1.0 ("Value")] -> w244
              frame "PWM" {
              }
              frame "Motor", Default {
              }
              frame "Analog Out" {
              }
            }
            n136 = property on="Motor" class="Clust (strict)"("Visible"=TRUE) -> ()  [unwired: 2 in, 2 out]
            n137 = property on="Value" class="Slide (strict)"("Value"=w245, "Scale.Minimum"=w247, "Scale.Maximum"=w246, "Scale.Increment"=w244) -> ()  [unwired: 2 in, 2 out]
            n138 = property on="On/Off" class="Bool (strict)"("Visible"=w249) -> ()  [unwired: 2 in, 2 out]
            n139 = property on="Test Slider" class="Slide (strict)"("Visible"=w249) -> ()  [unwired: 2 in, 2 out]
            n140 = property on="Test Ring" class="Ring (strict)"("Visible"=w249) -> ()  [unwired: 2 in, 2 out]
            n141 = property on="Rev/Fwd" class="Clust (strict)"("Visible"=w249) -> ()  [unwired: 2 in, 2 out]
          }
          frame "Servo" {
            w265 = FALSE ("Visible")
            n142 = call <vilib>:"NT Read Number.vi"("Name"=w267) -> ("Numeric"=w266:dbl)  [unwired: 9 in, 1 out]
            n143 = property on="Test Slider" class="Slide (strict)"("Visible"=TRUE, "Scale.Maximum"=170.0 ("Scale.Range:Maximum")) -> ()  [unwired: 2 in, 2 out]
            n144 = local write "Test Slider"(w266) -> ()
            n145 = property on="Motor" class="Clust (strict)"("Visible"=w265) -> ()  [unwired: 2 in, 2 out]
            n146 = property on="Rev/Fwd" class="Clust (strict)"("Visible"=w265) -> ()  [unwired: 2 in, 2 out]
            n147 = property on="On/Off" class="Bool (strict)"("Visible"=w265) -> ()  [unwired: 2 in, 2 out]
            n148 = property on="Test Ring" class="Ring (strict)"("Visible"=w265) -> ()  [unwired: 2 in, 2 out]
          }
          frame "Relay", "Solenoid" {
            w268 = FALSE ("Visible")
            n149 = property on="Motor" class="Clust (strict)"("Visible"=w268) -> ()  [unwired: 2 in, 2 out]
            n150 = property on="Test Slider" class="Slide (strict)"("Visible"=w268) -> ()  [unwired: 2 in, 2 out]
            n151 = Search and Replace String(input string=w269, search string="/Value  **", replace string="/Direction") -> (result string=w275:string)  [unwired: 5 in, 3 out]
            n152 = property on="Test Ring" class="Ring (strict)"("Visible"=w268) -> ()  [unwired: 2 in, 2 out]
            n153 = call <vilib>:"NT Read String.vi"("Name"=w275) -> ("String"=w273:string)  [unwired: 9 in, 1 out]
            n154 = Equal?(x="Both directions", y=w273) -> (x = y?=w271:bool)
            n155 = Not(x=w271) -> (.not. x?=w272:bool)
            n156 = property on="Rev/Fwd" class="Clust (strict)"("Visible"=w271) -> ()  [unwired: 2 in, 2 out]
            n157 = property on="On/Off" class="Bool (strict)"("Visible"=w272, "Caption.Text"=w270) -> ()  [unwired: 2 in, 2 out]
          }
          frame "Compressor", "Digital Out" {
            w278 = FALSE ("Visible")
            # "Get direction and finish"
            n158 = property on="Motor" class="Clust (strict)"("Visible"=w278) -> ()  [unwired: 2 in, 2 out]
            n159 = property on="Test Slider" class="Slide (strict)"("Visible"=w278) -> ()  [unwired: 2 in, 2 out]
            n160 = property on="Test Ring" class="Ring (strict)"("Visible"=w278) -> ()  [unwired: 2 in, 2 out]
            n161 = property on="On/Off" class="Bool (strict)"("Visible"=TRUE, "Caption.Text"=w279) -> ()  [unwired: 2 in, 2 out]
            n162 = property on="Rev/Fwd" class="Clust (strict)"("Visible"=FALSE) -> ()  [unwired: 2 in, 2 out]
          }
          frame "Camera" {
            n163 = call <vilib>:"Get Last Path Segment.vi"("String in"=w286) -> ("String out"=w287:string)  [unwired: 10 in]
            n164 = property on="On/Off" class="Bool (strict)"("Visible"=FALSE) -> ()  [unwired: 2 in, 2 out]
            n165 = property on="Motor" class="Clust (strict)"("Visible"=FALSE) -> ()  [unwired: 2 in, 2 out]
            n166 = property on="Rev/Fwd" class="Clust (strict)"("Visible"=FALSE) -> ()  [unwired: 2 in, 2 out]
            n167 = case shown="\"White Balance  **\"" w287 {
              tunnel: w286 -> [w293 w302 w311 w320 w329 _ w335]
              tunnel: w285 -> [w291 w299 w308 w317 w326 _ _]
              frame "Size  **" {
                n168 = Index Array(array=w291) -> (element=w290:cluster{string[]})  [unwired: 1 in]
                n169 = call <vilib>:"NT Read String.vi"("Name"=w293) -> ("String"=w292:string)  [unwired: 9 in, 1 out]
                n170 = Unbundle(w290) -> (w288:string[])
                n171 = Match First String(2:w288, 3:w292) -> (0:w289:i32)  [unwired: 1 out]
                n172 = property on="Test Ring" class="Ring (strict)"("Value"=w289, "Strings []"=w288) -> ()  [unwired: 2 in, 2 out]
                n173 = property on="Test Ring" class="Ring (strict)"("Visible"=TRUE) -> ()  [unwired: 2 in, 2 out]
                n174 = property on="Test Slider" class="Slide (strict)"("Visible"=FALSE) -> ()  [unwired: 2 in, 2 out]
              }
              frame "White Balance  **" {
                n175 = Index Array(array=w299, index=1) -> (element=w300:cluster{string[]})
                n176 = call <vilib>:"NT Read String.vi"("Name"=w302) -> ("String"=w301:string)  [unwired: 9 in, 1 out]
                n177 = Unbundle(w300) -> (w297:string[])
                n178 = Match First String(2:w297, 3:w301) -> (0:w296:i32)  [unwired: 1 out]
                n179 = property on="Test Ring" class="Ring (strict)"("Value"=w296, "Strings []"=w297) -> ()  [unwired: 2 in, 2 out]
                n180 = property on="Test Ring" class="Ring (strict)"("Visible"=TRUE) -> ()  [unwired: 2 in, 2 out]
                n181 = property on="Test Slider" class="Slide (strict)"("Visible"=FALSE) -> ()  [unwired: 2 in, 2 out]
              }
              frame "Exposure  **" {
                n182 = Index Array(array=w308, index=2) -> (element=w309:cluster{string[]})
                n183 = call <vilib>:"NT Read String.vi"("Name"=w311) -> ("String"=w310:string)  [unwired: 9 in, 1 out]
                n184 = Unbundle(w309) -> (w305:string[])
                n185 = Match First String(2:w305, 3:w310) -> (0:w306:i32)  [unwired: 1 out]
                n186 = property on="Test Ring" class="Ring (strict)"("Value"=w306, "Strings []"=w305) -> ()  [unwired: 2 in, 2 out]
                n187 = property on="Test Ring" class="Ring (strict)"("Visible"=TRUE) -> ()  [unwired: 2 in, 2 out]
                n188 = property on="Test Slider" class="Slide (strict)"("Visible"=FALSE) -> ()  [unwired: 2 in, 2 out]
              }
              frame "Exposure Priority  **" {
                n189 = Index Array(array=w317, index=3) -> (element=w318:cluster{string[]})
                n190 = call <vilib>:"NT Read String.vi"("Name"=w320) -> ("String"=w319:string)  [unwired: 9 in, 1 out]
                n191 = Unbundle(w318) -> (w314:string[])
                n192 = Match First String(2:w314, 3:w319) -> (0:w315:i32)  [unwired: 1 out]
                n193 = property on="Test Ring" class="Ring (strict)"("Value"=w315, "Strings []"=w314) -> ()  [unwired: 2 in, 2 out]
                n194 = property on="Test Ring" class="Ring (strict)"("Visible"=TRUE) -> ()  [unwired: 2 in, 2 out]
                n195 = property on="Test Slider" class="Slide (strict)"("Visible"=FALSE) -> ()  [unwired: 2 in, 2 out]
              }
              frame "Color Enable  **" {
                n196 = Index Array(array=w326, index=4) -> (element=w327:cluster{string[]})
                n197 = call <vilib>:"NT Read String.vi"("Name"=w329) -> ("String"=w328:string)  [unwired: 9 in, 1 out]
                n198 = Unbundle(w327) -> (w323:string[])
                n199 = Match First String(2:w323, 3:w328) -> (0:w324:i32)  [unwired: 1 out]
                n200 = property on="Test Ring" class="Ring (strict)"("Value"=w324, "Strings []"=w323) -> ()  [unwired: 2 in, 2 out]
                n201 = property on="Test Ring" class="Ring (strict)"("Visible"=TRUE) -> ()  [unwired: 2 in, 2 out]
                n202 = property on="Test Slider" class="Slide (strict)"("Visible"=FALSE) -> ()  [unwired: 2 in, 2 out]
              }
              frame Default {
                n203 = property on="Test Ring" class="Ring (strict)"("Visible"=FALSE) -> ()  [unwired: 2 in, 2 out]
                n204 = property on="Test Slider" class="Slide (strict)"("Visible"=FALSE) -> ()  [unwired: 2 in, 2 out]
              }
              frame "Brightness  **", "Color Level  **", "Compression  **", "FPS  **", "Sharpness  **" {
                n205 = call <vilib>:"NT Read Number.vi"("Name"=w335) -> ("Numeric"=w334:dbl)  [unwired: 9 in, 1 out]
                n206 = local write "Test Slider"(w334) -> ()
                n207 = property on="Test Slider" class="Slide (strict)"("Visible"=TRUE, "Scale.Maximum"=100.0 ("Scale.Range:Maximum")) -> ()  [unwired: 2 in, 2 out]
                n208 = property on="Test Ring" class="Ring (strict)"("Visible"=FALSE) -> ()  [unwired: 2 in, 2 out]
              }
            }
          }
        }
        n209 = property on="Progress" class="Clust (strict)"("Visible"=FALSE) -> ()  [unwired: 2 in, 2 out]
      }
      event "Test Name": Mouse Enter {
        # "Populate the ring with the list of tests"
        n210 = event-data() -> ()  [unwired: 1 in, 1 out]
        n211 = call <vilib>:"NT Read String Array.vi"("Name"="/TestMode/TestList") -> ("String Array"=w343:string[])  [unwired: 9 in, 1 out]
        n212 = Build Array (concatenate)("Select the test to run...", w343) -> (w342:string[])
        n213 = property on="Test Name" class="Ring (strict)"("Strings []"=w342) -> ()  [unwired: 2 in, 2 out]
      }
      event "Test Name": Value Change {
        w345 = FALSE ("Visible")
        # "Tell the robot the test name to run"
        n214 = event-data() -> ("NewVal"=w349:u16)  [unwired: 1 in]
        n215 = property on="Test Name" class="Ring (strict)"() -> ("Strings []"=w350:string[])  [unwired: 2 in, 2 out]
        n216 = local write "Progress"(T6 {"Test Progress"=0, "Test Progress Text"=""} ("Progress")) -> ()
        n217 = Index Array(array=w350, index=w349) -> (element=w348:string)
        n218 = call <vilib>:"NT Write String.vi"("String"=w348, "Name"="/TestMode/TestName") -> ()  [unwired: 9 in, 1 out]
        n219 = property on="Progress" class="Clust (strict)"("Visible"=TRUE) -> ()  [unwired: 2 in, 2 out]
        n220 = property on="Motor" class="Clust (strict)"("Visible"=w345) -> ()  [unwired: 2 in, 2 out]
        n221 = property on="Test Slider" class="Slide (strict)"("Visible"=w345) -> ()  [unwired: 2 in, 2 out]
        n222 = property on="On/Off" class="Bool (strict)"("Visible"=w345) -> ()  [unwired: 2 in, 2 out]
        n223 = property on="Rev/Fwd" class="Clust (strict)"("Visible"=w345) -> ()  [unwired: 2 in, 2 out]
        n224 = property on="Test Ring" class="Ring (strict)"("Visible"=w345) -> ()  [unwired: 2 in, 2 out]
      }
      event "Select Auto": Mouse Enter {
        # "Populate the combo box with the list of autonomous options"
        n225 = event-data() -> ()  [unwired: 1 in, 1 out]
        n226 = call <vilib>:"NT Read String Array.vi"("Name"="Auto List") -> ("String Array"=w352:string[])  [unwired: 9 in, 1 out]
        n227 = property on="Select Auto" class="CmbBox"("Strings[]"=w352) -> ()  [unwired: 2 in, 2 out]
      }
      event "Select Auto": Value Change {
        # "User modified the Auto Selection. Write to NT variable so robot knows."
        n228 = event-data() -> ("NewVal"=w355:string)  [unwired: 1 in]
        n229 = call <vilib>:"NT Write String.vi"("String"=w355, "Name"="Auto Selector") -> ()  [unwired: 9 in, 1 out]
      }
      event "Command Selection": Value Change {
        # "Get the params and show in table"
        n230 = event-data() -> ("NewVal"=w361:i32)  [unwired: 1 in]
        n231 = property on="Command Selection" class="MCListbox (strict)"() -> ("ItemNames"=w359:string[][])  [unwired: 2 in, 2 out]
        n232 = call <vilib>:"WPI_DashboardUpdate Command Params.vi"("NewVal"=w361, "Commands"=w359, "Param Tbl"=w360) -> ()  [unwired: 8 in, 1 out]
      }
      event "Execute Command": Value Change {
        # "Started one, Unique ID holds\nresponse"
        n233 = event-data() -> ()  [unwired: 1 in, 1 out]
        n234 = property on="Command Selection" class="MCListbox (strict)"() -> ("ItemNames"=w372:string[][])  [unwired: 2 in, 2 out]
        n235 = Index Array(array=w372, index (row)="Command Selection", index (col)=0) -> (element=w370:string)
        n236 = call <vilib>:"Invoke Commands.vi"("Command Params"="Command Params", "Function Name"=w370) -> ("Params"=w366:u8, "Started"=w365:bool)  [unwired: 7 in, 1 out]
        n237 = Array Subset(array="Command Params", length (row)=w366) -> (w367:string[][])  [unwired: 3 in]
        n238 = Select(t="Executing" ("Cmd Status"), s=w365, f="" ("Cmd Status")) -> (s? t:f=→"Cmd Status":string)
      }
      event "Command Selection": Double Click {
        n239 = event-data() -> ("Row"=w380:i32)  [unwired: 1 in]
        n240 = property on="Command Selection" class="MCListbox (strict)"() -> ("ItemNames"=w383:string[][])  [unwired: 2 in, 2 out]
        n241 = local read "Command Params"() -> (w379:string[][])
        n242 = Index Array(array=w383, index (row)=w380, index (col)=0) -> (element=w381:string)
        n243 = call <vilib>:"Invoke Commands.vi"("Command Params"=w379, "Function Name"=w381) -> ("Params"=w378:u8, "Started"=w373:bool)  [unwired: 7 in, 1 out]
        n244 = Array Subset(array=w379, length (row)=w378) -> (w377:string[][])  [unwired: 3 in]
        n245 = Select(t="Executing" ("Cmd Status"), s=w373, f="" ("Cmd Status")) -> (s? t:f=w374:string)
        n246 = local write "Cmd Status"(w374) -> ()
      }
      event "CheckList": Double Click {
        # "Shift clears all"
        # "Update symbols on the listbox"
        n247 = event-data() -> ("PlatMods.Shift"=w385:bool, "Row"=w387:i32)  [unwired: 1 in]
        n248 = case shown="True" w385 {
          tunnel: w387 -> [w391 _]
          tunnel: 1 -> [w390 _]
          frame False {
            n249 = property on="CheckList" class="LstBox (strict)"() -> ("Item Symbols"=w389:i32[])  [unwired: 2 in, 2 out]
            n250 = Replace Array Subset(array=w389, new element=w390, index=w391) -> (w388:i32[])
            n251 = property on="CheckList" class="LstBox (strict)"("Item Symbols"=w388) -> ()  [unwired: 2 in, 2 out]
          }
          frame True {
            w392 = 0 ("Top Row")
            n252 = property on="CheckList" class="LstBox (strict)"() -> ("Number of Rows"=w394:u32)  [unwired: 2 in, 2 out]
            n253 = Initialize Array(0, w394) -> (w393:i32[])
            n254 = property on="CheckList" class="LstBox (strict)"("Top Row"=w392, "Value"=w392, "Item Symbols"=w393) -> ()  [unwired: 2 in, 2 out]
          }
        }
      }
      event "CheckList": Key Down {
        # "Update symbols on the listbox\nLeft and right keys check and uncheck"
        n255 = event-data() -> ("VKey"=w398:T19)  [unwired: 1 in]
        n256 = case shown="\"Left\", \"Right\"" w398 {
          selector: w398 -> [w403 _]
          tunnel: eventvkey."Left" ("VKey") -> [w401 _]
          frame "Left", "Right" {
            n257 = Equal?(x=w401, y=w403) -> (x = y?=w402:bool)
            n258 = Select(t=0, s=w402, f=1) -> (s? t:f=w404:i32)
            n259 = property on="CheckList" class="LstBox (strict)"() -> ("Item Symbols"=w407:i32[])  [unwired: 2 in, 2 out]
            n260 = Replace Array Subset(array=w407, new element=w404, index="CheckList") -> (w406:i32[])
            n261 = property on="CheckList" class="LstBox (strict)"("Item Symbols"=w406) -> ()  [unwired: 2 in, 2 out]
          }
          frame Default {
          }
        }
      }
      event "Motor.Enable": Value Change {
        # "When the test mode otor enable helper is set, update that\ntree row item's value"
        n262 = event-data() -> ("NewVal"=w413:bool)  [unwired: 1 in]
        n263 = Unbundle("Motor") -> ("Value"=w412:dbl)  [unwired: 1 out]
        n264 = Select(t=w412, s=w413, f=0.0) -> (s? t:f=w410:dbl)
        n265 = call <vilib>:"NT Write Number.vi"("Numeric"=w410, "Name"=w409) -> ()  [unwired: 9 in, 1 out]
      }
      event "Test Slider": Value Change {
        # "When the test mode slider helper is set, update that\ntree row item's value"
        n266 = event-data() -> ("NewVal"=w416:dbl)  [unwired: 1 in]
        n267 = call <vilib>:"NT Write Number.vi"("Numeric"=w416, "Name"=w417) -> ()  [unwired: 9 in, 1 out]
      }
      event "On/Off": Value Change {
        # "When the test mode on/off helper value is set, update that\ntree row item's value"
        n268 = event-data() -> ("NewVal"=w421:bool)  [unwired: 1 in]
        n269 = Boolean To (0,1)(Boolean=w421) -> (0, 1=w420:i16)
        n270 = call <vilib>:"NT Write Number.vi"("Numeric"=w420, "Name"=w419) -> ()  [unwired: 9 in, 1 out]
      }
      event "Rev/Fwd": Value Change {
        # "When the test mode helper value for relays is set, update that\ntree row item's value"
        n271 = event-data() -> ("NewVal.Forward"=w429:bool, "NewVal.Reverse"=w428:bool)  [unwired: 1 in]
        n272 = Boolean To (0,1)(Boolean=w429) -> (0, 1=w425:i16)
        n273 = Boolean To (0,1)(Boolean=w428) -> (0, 1=w427:i16)
        n274 = Negate(x=w427) -> (-x=w426:i16)
        n275 = Add(x=w425, y=w426) -> (x+y=w424:i16)
        n276 = call <vilib>:"NT Write Number.vi"("Numeric"=w424, "Name"=w423) -> ()  [unwired: 9 in, 1 out]
      }
      event "Test Ring": Value Change {
        # "When a test mode helper value is selected from the ring,\nset the tree item's variable to the string value"
        n277 = event-data() -> ("NewVal"=w433:u16)  [unwired: 1 in]
        n278 = property on="Test Ring" class="Ring (strict)"() -> ("Strings []"=w434:string[])  [unwired: 2 in, 2 out]
        n279 = Index Array(array=w434, index=w433) -> (element=w432:string)
        n280 = call <vilib>:"NT Write String.vi"("String"=w432, "Name"=w431) -> ()  [unwired: 9 in, 1 out]
      }
      event "Rec Mode": Value Change {
        # "Update globals for recording mode and path to read log from.\nClear when logging and let NetworkTables set path for vision to\nuse."
        n281 = event-data() -> ("NewVal"=w445:enum32{"Stop", "Record", "Playback"})  [unwired: 1 in]
        n282 = global write "WPI_DashboardLogging Global.vi" "Logging Filename"(path "") -> ()
        n283 = global write "WPI_DashboardLogging Global.vi" "Recording"(w445) -> ()
        n284 = case shown="\"Playback\"" w445 {
          tunnel: w444 -> [_ w447 w456]
          tunnel: [_ _ w455] -> w442
          tunnel: [_ _ w454] -> _
          tunnel: w440 -> [_ _ w452]
          tunnel: cluster{i32, i32} {-250, 170} -> [_ _ w451]
          tunnel: [_ _ T20 {"Image Size"=TRUE, "Image Type"=TRUE, "Pixel Value"=TRUE, "ROI Information"=TRUE, "Zoom Factor"=FALSE} ("Image Information Shown:All Elements")] -> w438
          tunnel: [_ _ TRUE ("Zoom Factor")] -> w437
          tunnel: w436 -> [_ _ w448]
          frame Default {
          }
          frame "Stop", "Record" {
            # "Place Window too"
            n285 = invoke class="VI" method="FP.Close"(reference=w447) -> (reference out=w446:refnum<vi>)  [unwired: 2 in, 2 out]
            n286 = invoke class="VI" method="Abort VI"(reference=w446) -> ()  [unwired: 2 in, 3 out]
          }
          frame "Playback" {
            n287 = call "Open Playback Panel.vi"("Offset"=w451, "DB VI Ref"=w452, "Playback in"=w456) -> ("Playback out"=w453:refnum<vi>)  [unwired: 8 in]
            n288 = register-events(w453, w448) -> (reference out=w455:refnum<event-registration>, error out=w454:errorcluster)  [unwired: 2 in]
          }
        }
        n289 = property on="Camera Image" class="ImageControl"("Image Information Shown"=w438, "Image Information Visible"=w437) -> ()  [unwired: 2 in, 2 out]
        n290 = call <vilib>:"WPI_DashboardNT Log FieldName Cache.vi"("Operation"=enum16{"Lookup/Add", "Index", "Clear"}."Clear") -> ()  [unwired: 8 in, 3 out]
      }
      event Panel Close {
        w458 = enum32{"Stop", "Record", "Playback"}."Stop" ("Rec Mode")
        # "Playback window has been closed, abort"
        n291 = event-data() -> ()  [unwired: 1 in, 4 out]
        n292 = local write "Rec Mode"(w458) -> ()
        n293 = global write "WPI_DashboardLogging Global.vi" "Recording"(w458) -> ()
      }
      event Panel Close {
        # "Abort playback window and ourself"
        n294 = event-data() -> ()  [unwired: 1 in, 4 out]
        n295 = invoke class="VI" method="FP.Close"(reference=w462) -> (reference out=w461:refnum<vi>)  [unwired: 2 in, 2 out]
        n296 = invoke class="VI" method="Abort VI"(reference=w461) -> (error out=w460:errorcluster)  [unwired: 2 in, 2 out]
        n297 = invoke class="VI" method="Abort VI"(error in=w460) -> ()  [unwired: 2 in, 3 out]
      }
      event User Event {
        n298 = event-data() -> ("IDs"=w469:cluster{"RPC field ID":u16, "Unique ID":u16}, "String"=w468:string)  [unwired: 1 in]
        n299 = Bundle("IDs"=w469, "String"=w468) -> (w467:T8)  [unwired: 1 in]
        n300 = call <vilib>:"Retrieve RPC Response.vi"("RPC Response"=w467) -> ("Output"=w465:string[][])  [unwired: 10 in]
        n301 = Build Array (concatenate)(w463, w465) -> (w464:string[][])
        n302 = local write "Command Params"(w464) -> ()
        n303 = local write "Cmd Status"("" ("Cmd Status")) -> ()
      }
      event "Tree": Double Click {
        n304 = event-data() -> ("PlatMods"=w473:T23, "Tag"=w472:string)  [unwired: 1 in]
        n305 = Unbundle(w473) -> ("Shift"=w471:bool)  [unwired: 4 out]
        n306 = Not(x=w471) -> (.not. x?=w470:bool)
        n307 = call <vilib>:"NT Update Persistence.vi"("Persistence"=w470, "Name"=w472) -> ()  [unwired: 9 in, 1 out]
      }
    }
  }
  n308 = while {
    tunnel: w64 -> [w476]
    i -> [w479]
    stop <- FALSE stop-if-true
    n309 = Wait (ms)(milliseconds to wait=u32 100) -> ()  [unwired: 1 out]
    n310 = case shown="\"Playback\"" "Rec Mode" {
      tunnel: w479 -> [_ _ w494]
      tunnel: [u32 2829099 ("Base Color") u32 11141120 ("Target Color") w483] -> w475
      frame "Stop", Default {
        # "Reset the color, extra updates don't cost much"
      }
      frame "Record" {
      }
      frame "Playback" {
        # "Playback"
        n311 = Quotient & Remainder(x=w494, y=u32 50 ("milliseconds to wait")) -> (x-y*floor(x/y)=w490:u32)  [unwired: 1 out]
        n312 = Divide(x=w490, y=u32 50 ("milliseconds to wait")) -> (x/y=w487:dbl)
        n313 = Multiply(x=6.283185307179586, y=w487) -> (x*y=w492:dbl)
        n314 = Sine(x=w492) -> (sin(x)=w491:dbl)
        n315 = Absolute Value(x=w491) -> (abs(x)=w484:dbl)
        n316 = call "Interpolate RGB Color.vi"("Proportion"=w484, "Target Color"=u32 30976, "Base Color"=u32 2829099) -> ("Result Color"=w483:u32)  [unwired: 8 in]
      }
    }
    n317 = property class="Pane"(reference=w476, "PaneColor"=w475) -> ()  [unwired: 1 in, 2 out]
  }
  n318 = local write "Dashboard Tab"(T2."Drive" ("Dashboard Tab")) -> ()
  n319 = property on="On/Off" class="Bool (strict)"("Visible"=w34) -> ()  [unwired: 2 in, 2 out]
  n320 = property on="Motor" class="Clust (strict)"("Visible"=w34) -> ()  [unwired: 2 in, 2 out]
  n321 = property on="Progress" class="Clust (strict)"("Visible"=w34) -> ()  [unwired: 2 in, 2 out]
  n322 = property on="Test Ring" class="Ring (strict)"("Visible"=w34) -> ()  [unwired: 2 in, 2 out]
  n323 = property on="Rev/Fwd" class="Clust (strict)"("Visible"=w34) -> ()  [unwired: 2 in, 2 out]
  n324 = while {
    tunnel: u16 1741 ("timeout ms (25000)") -> [w496]
    stop <- FALSE stop-if-true
    n325 = TCP Create Listener(10:w496) -> (0:w495:errorcluster, 3:w497:refnum<k5>)  [unwired: 4 in, 1 out]
    n326 = case shown="No Error" w495 {
      selector: w495 -> [w499 _]
      tunnel: w497 -> [w500 _]
      frame No Error {
        n327 = while {
          tunnel: w500 -> [w503]
          tunnel: w499 -> [w502]
          stop <- FALSE stop-if-true
          n328 = TCP Wait On Listener(8:w502, 11:w503) -> (0:w504:errorcluster, 4:w505:refnum<k5>)  [unwired: 2 in, 3 out]
          n329 = local write "TCP"(w505) -> ()
          n330 = case shown="No Error" w504 {
            frame No Error {
            }
            frame Error {
              n331 = Wait (ms)(milliseconds to wait=u32 1000) -> ()  [unwired: 1 out]
            }
          }
        }
      }
      frame Error {
        n332 = Wait (ms)(milliseconds to wait=u32 1000) -> ()  [unwired: 1 out]
      }
    }
  }
  n333 = local write "Command Selection"(u16 0 ("milliseconds to wait")) -> ()
  n334 = local write "Command Params"(string[][] [] ("Command Params")) -> ()
  n335 = global write "WPI_DashboardLogging Global.vi" "Recording"(w58) -> ()
  n336 = local write "Rec Mode"(w58) -> ()
  n337 = call <vilib>:"NT Write String.vi"("String"="Select Auto", "Name"="Auto Selector") -> ()  [unwired: 9 in, 1 out]
